vi "MoveBySteps.vi"(6 "Direction":enum16{"Forward", "Backwards"}(ring), 7 "Polarity":enum16{"Positive", "Negative"}(ring), 8 "error in (no error)":errorcluster, 9 "Speed":u32, 10 "Steps":enum32{""}(ring), 11 "TranslationStage in":refnum<class "TranslationStagesInterface.lvclass">) -> (0 "error out":errorcluster, 3 "TranslationStage out":refnum<class "TranslationStagesInterface.lvclass">)   [LabVIEW 2023, in "TranslationStagesInterface.lvclass"]
uses:
  TranslationStagesInterface.lvclass
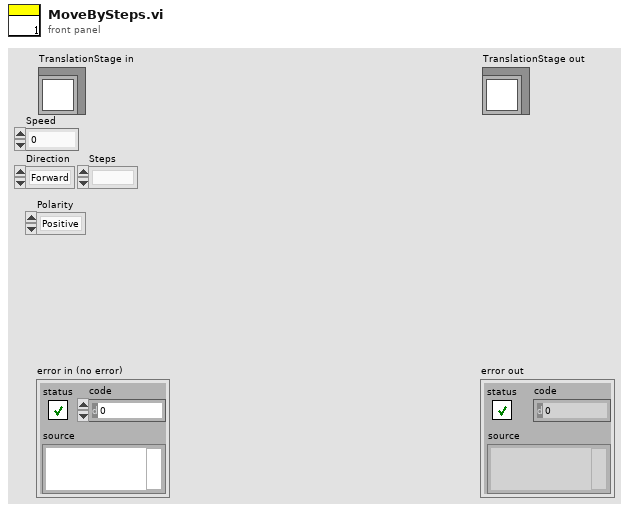
[diagram p1: front panel]
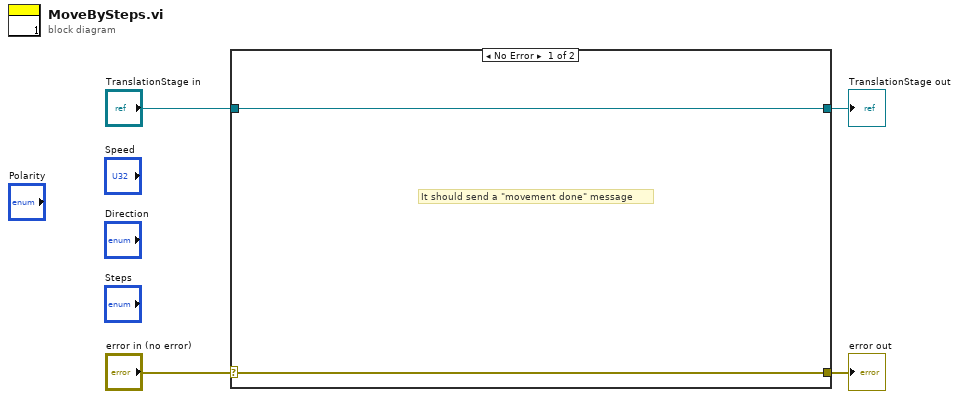
[diagram p0: block diagram]
diagram:
  n1 = case shown="No Error" "error in (no error)" {
    selector: "error in (no error)" -> [w5 w8]
    tunnel: [w5 w8] -> w3
    tunnel: [w6 w7] -> w1
    tunnel: "TranslationStage in" -> [w6 w7]
    frame No Error {
      # "It should send a \"movement done\" message"
    }
    frame Error {
    }
  }
  "error out" <- w3
  "TranslationStage out" <- w1
